vi "ReadBackHNSLogsV2.vi"() -> ()   [LabVIEW 2014]
uses:
  SABL_Source_OLD/HNSCluster.ctl
  SABL_Source_OLD/HNSAI.ctl
  SABL_Source_OLD/HNSWarnings.ctl
  SABL_Source_OLD/HNSMetaCluster.ctl
panel:
  out "appended array":T1[](array[typedef]) {"Overall Status" format="%x"; "PEP Request Word 2" format="%x"; "PEP Request Word 1" format="%x"}
  in  "Array 4":T1[](array[typedef])=array[14302 elements] {"Overall Status" format="%x"; "PEP Request Word 2" format="%x"; "PEP Request Word 1" format="%x"}
  out "Array 3":T2[](array[typedef])
  in  "Array 2":T2[](array[typedef])=array[38192 elements]
  out "Numeric 6":i32
  out "Numeric 5":i32
  out "status 2":bool
  out "Numeric 4":i32
  out "length 2":i32
  in  "HNSLog-2016-02-24-13-03-37.log":T2[](array[typedef])=array[25394 elements]
  out "length":i32
  out "status":bool
  out "Numeric 3":i32
  out "Array":T2[](array[typedef])
  out "transposed array":dbl[][](array[numeric])
  out "Number of Files":i32
  out "All Files in Dir":path[](array[path])
  out "Numeric 2":i32
  out "Numeric":i32
  out "Waveform Graph":dbl[][](graph)
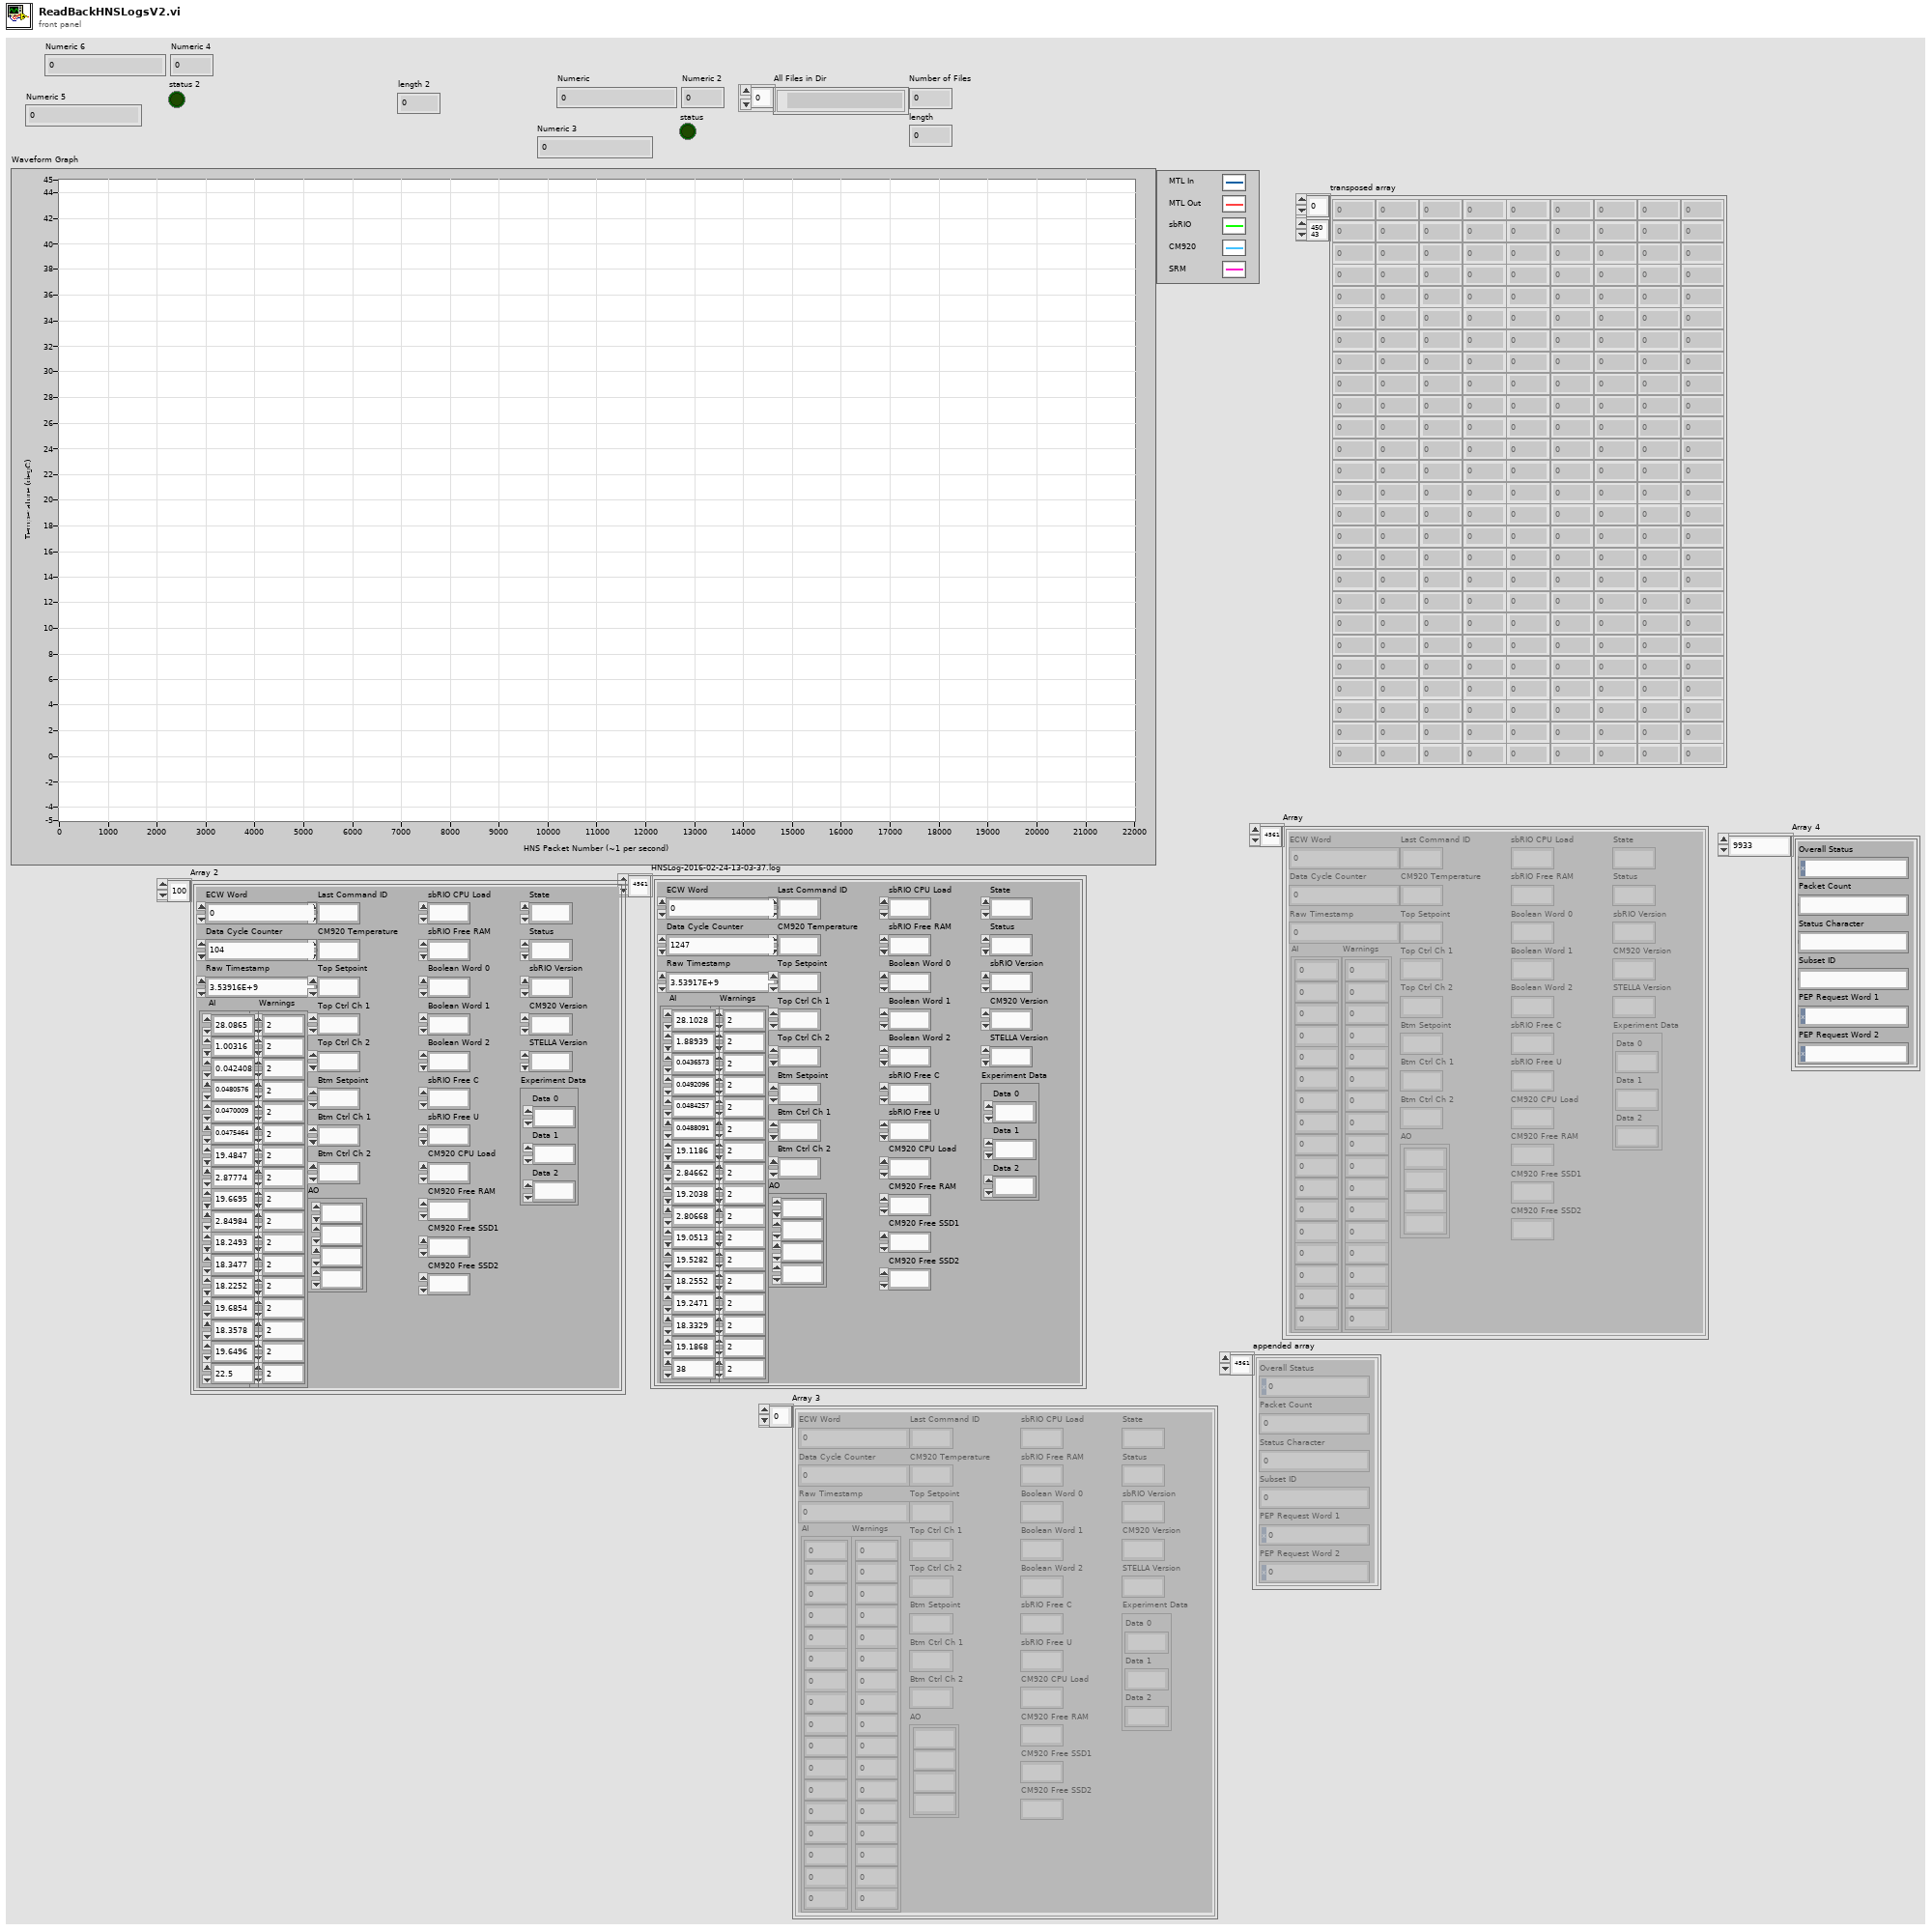
[diagram p1: front panel]
types:
  T1 = typedef "HNSMetaCluster.ctl" = cluster{"Overall Status":u32, "Packet Count":u32, "Status Character":u8, "Subset ID":u16, "PEP Request Word 1":u16, "PEP Request Word 2":u16}
  T2 = typedef "HNSCluster.ctl" = cluster{"ECW Word":u16, "Data Cycle Counter":u16, "Raw Timestamp":dbl, "AI":T3, "Warnings":T4, "Last Command ID":u8, "CM920 Temperature":sgl, "Top Setpoint":sgl, "Top Ctrl Ch 1":i16, "Top Ctrl Ch 2":i16, "Btm Setpoint":sgl, "Btm Ctrl Ch 1":i16, "Btm Ctrl Ch 2":i16, "AO":cluster{sgl, sgl, sgl, sgl}, "sbRIO CPU Load":i16, "sbRIO Free RAM":i16, "Boolean Word 0":i16, "Boolean Word 1":i16, "Boolean Word 2":i16, "sbRIO Free C":i16, "sbRIO Free U":i16, "CM920 CPU Load":i16, "CM920 Free RAM":i16, "CM920 Free SSD1":i16, "CM920 Free SSD2":i16, "State":i16, "Status":i16, "sbRIO Version":sgl, "CM920 Version":sgl, "STELLA Version":sgl, "Experiment Data":cluster{"Data 0":sgl, "Data 1":sgl, "Data 2":sgl}}
  T3 = typedef "HNSAI.ctl" = cluster{"AI0 - Payload Voltage":sgl, "AI1 - Payload Current":sgl, "AI2 - SRM AI1":sgl, "AI3 - SRM AI2":sgl, "AI4 - SRM AI3":sgl, "AI5 - SRM AI4":sgl, "AI6 - Top Back Temp":sgl, "AI7 - Top TEC Current":sgl, "AI8 - Btm Back Temp":sgl, "AI9 - Btm TEC Current":sgl, "AI10 - MTL In Temp":sgl, "AI11 - MTL Out Temp":sgl, "AI12 - Top HX Temp":sgl, "AI13 - Top Front Temp":sgl, "AI14 - Btm HX Temp":sgl, "AI15 - Btm Front Temp":sgl, "AIBT - sbRIO Temp":sgl}
  T4 = typedef "HNSWarnings.ctl" = cluster{"AI0 Warning - Payload Voltage":i8, "AI1 Warning- Payload Current":i8, "AI2 Warning - SRM AI1":i8, "AI3 Warning - SRM AI2":i8, "AI4 Warning - SRM AI3":i8, "AI5 Warning - SRM AI4":i8, "AI6 Warning - Top Back Temp":i8, "AI7 Warning - Top TEC Current":i8, "AI 8 Warning - Btm Back Temp":i8, "AI9 Warning - Btm TEC Current":i8, "AI10 Warning - MTL In Temp":i8, "AI11 Warning - MTL Out Temp":i8, "AI12 Warning - Top HX Temp":i8, "AI13 Warning - Top Front Temp":i8, "AI14 Warning - Btm HX Temp":i8, "AI15 Warning - Btm Front Temp":i8, "AIBT Warning - sbRIO Temp":i8}
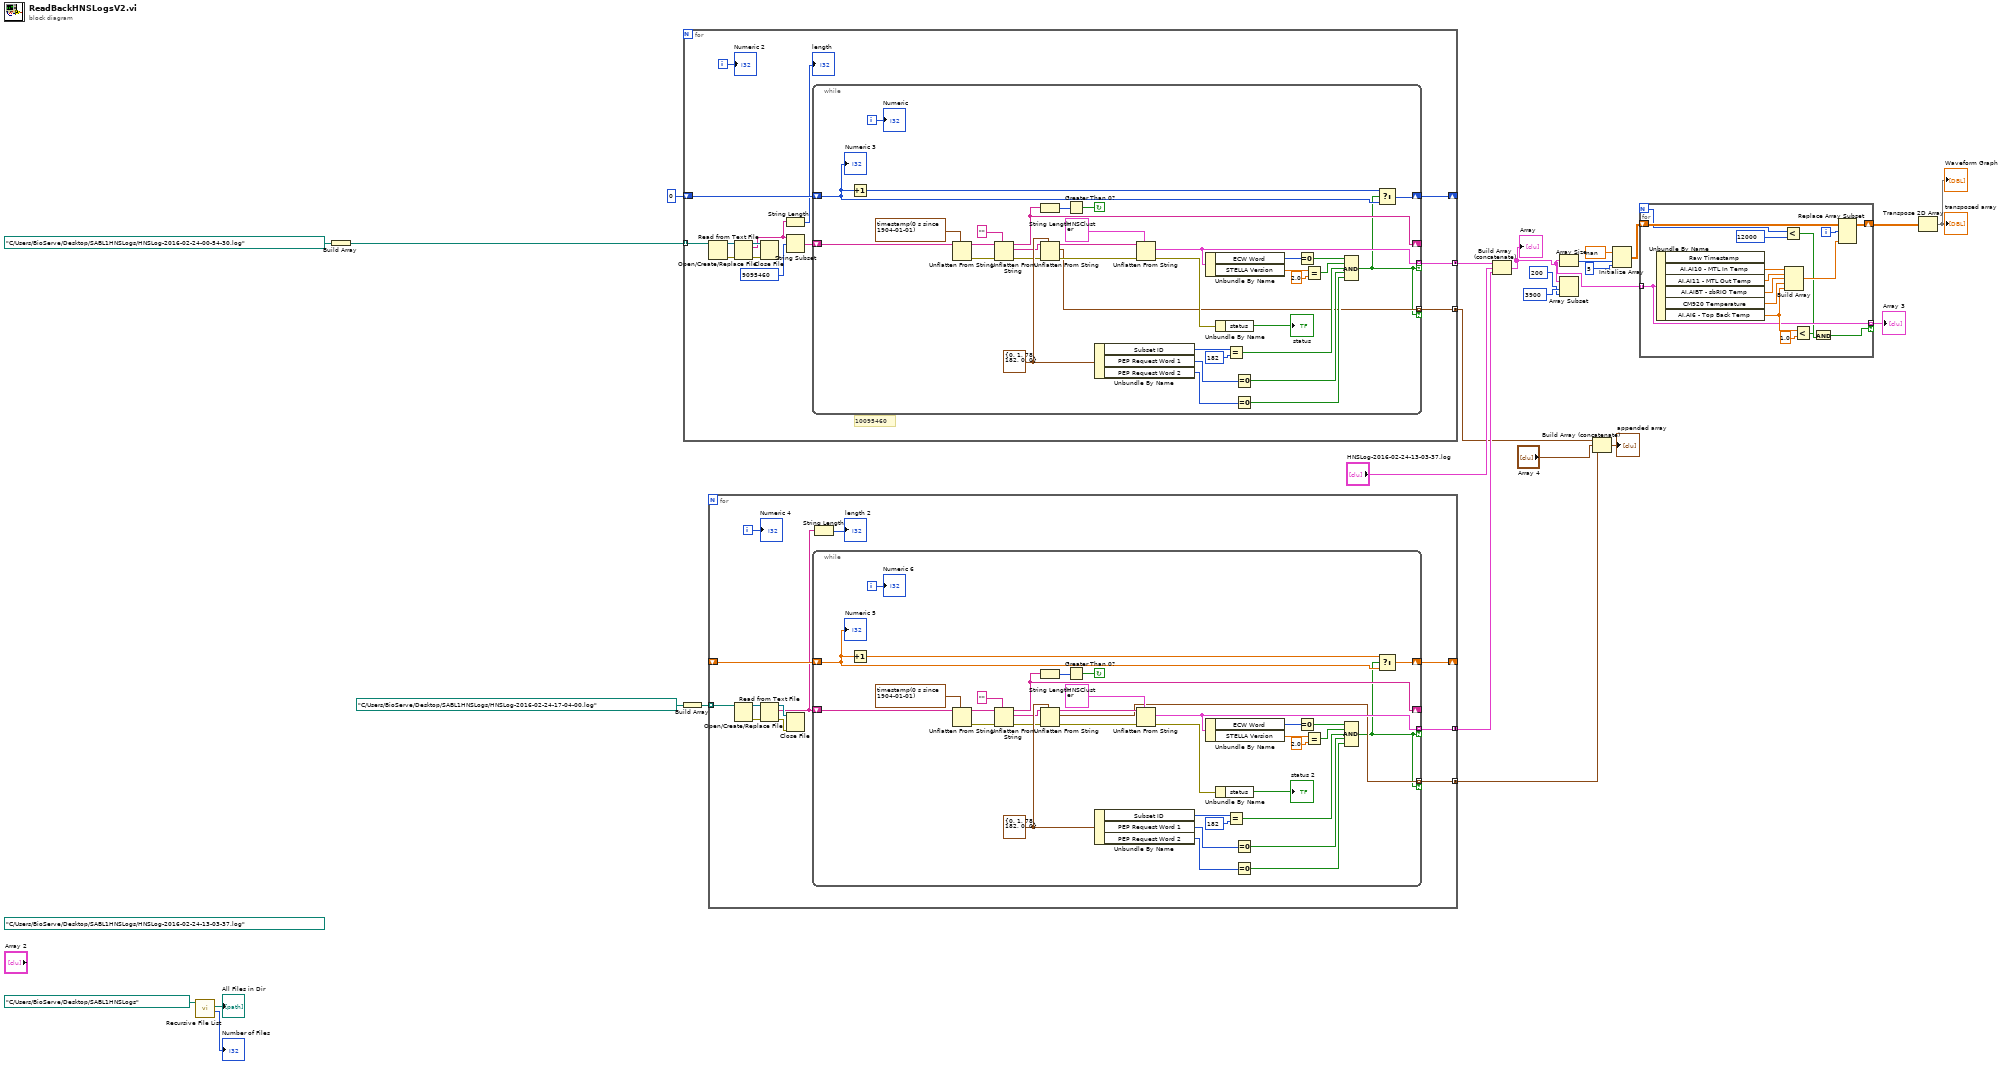
[diagram p0: block diagram]
diagram:
  (unwired) path "C:/Users/BioServe/Desktop/SABL1HNSLogs/HNSLog-2016-02-24-13-03-37.log" ("Folder Path")
  n1 = call <vilib>:"Recursive File List.vi"("Folder Path"=path "C:/Users/BioServe/Desktop/SABL1HNSLogs") -> ("Number of Files"=→"Number of Files":i32, "All Files in Dir"=→"All Files in Dir":path[])  [unwired: 6 in, 3 out]
  n2 = Build Array(path "C:/Users/BioServe/Desktop/SABL1HNSLogs/HNSLog-2016-02-24-00-54-30.log" ("Folder Path")) -> (w15:path[])
  n3 = for {
    tunnel: w15 -> [w31] mode=indexing
    tunnel: [w34] -> w13 mode=concatenating
    shift-right: [w32] -> _
    shift-left: 0 -> [w33]
    tunnel: [w26] -> w5 mode=concatenating
    i -> [w35]
    # "10095460"
    n4 = Open/Create/Replace File(file path (use dialog)=w31) -> (refnum out=w39:refnum<file>, error out=w38:errorcluster)  [unwired: 5 in, 1 out]
    n5 = Read from Text File(file (use dialog)=w39, error in=w38) -> (refnum out=w36:refnum<file>, text=w29:string, error out=w37:errorcluster)  [unwired: 2 in, 1 out]
    n6 = Close File(refnum=w36, error in=w37) -> ()  [unwired: 2 out]
    n7 = String Length(string=w29) -> (length=→"length":i32)
    n8 = String Subset(string=w29, offset (0)=9095460) -> (substring=w28:string)  [unwired: 1 in]
    n9 = while {
      tunnel: [w71] -> w34 mode=indexing if=w40
      shift-right: [w42] -> _
      shift-left: w28 -> [w54]
      shift-right: [w63] -> w32
      shift-left: w33 -> [w64]
      tunnel: [w41] -> w26 mode=indexing if=w40
      i -> [w73]
      stop <- w66 continue-if-true
      w62 = T1 {"Overall Status"=0, "Packet Count"=1, "Status Character"=78, "Subset ID"=182, "PEP Request Word 1"=0, "PEP Request Word 2"=0} ("HNS Meta Cluster")
      n10 = Increment(x=w64) -> (x+1=w65:i32)
      n11 = Unflatten From String(type=timestamp(0 s since 1904-01-01), binary string=w54) -> (rest of the binary string=w47:string, error out=w45:errorcluster)  [unwired: 3 in, 1 out]
      n12 = Unflatten From String(type="", binary string=w47, error in (no error)=w45) -> (rest of the binary string=w42:string, value=w46:string, error out=w44:errorcluster)  [unwired: 2 in]
      n13 = String Length(string=w42) -> (length=w67:i32)
      n14 = Unflatten From String(type=w62, binary string=w46, error in (no error)=w44) -> (rest of the binary string=w72:string, value=w41:T1, error out=w43:errorcluster)  [unwired: 2 in]
      n15 = Greater Than 0?(x=w67) -> (x > 0?=w66:bool)
      n16 = Unbundle By Name(w62) -> ("Subset ID"=w61:u16, "PEP Request Word 1"=w58:u16, "PEP Request Word 2"=w55:u16)
      n17 = Unflatten From String(type=T2 {"ECW Word"=0, "Data Cycle Counter"=0, "Raw Timestamp"=0.0, "AI"={"AI0 - Payload Voltage"=0.0, "AI1 - Payload Current"=0.0, "AI2 - SRM AI1"=0.0, "AI3 - SRM AI2"=0.0, "AI4 - SRM AI3"=0.0, "AI5 - SRM AI4"=0.0, "AI6 - Top Back Temp"=0.0, "AI7 - Top TEC Current"=0.0, "AI8 - Btm Back Temp"=0.0, "AI9 - Btm TEC Current"=0.0, "AI10 - MTL In Temp"=0.0, "AI11 - MTL Out Temp"=0.0, "AI12 - Top HX Temp"=0.0, "AI13 - Top Front Temp"=0.0, "AI14 - Btm HX Temp"=0.0, "AI15 - Btm Front Temp"=0.0, "AIBT - sbRIO Temp"=0.0}, "Warnings"={"AI0 Warning - Payload Voltage"=0, "AI1 Warning- Payload Current"=0, "AI2 Warning - SRM AI1"=0, "AI3 Warning - SRM AI2"=0, "AI4 Warning - SRM AI3"=0, "AI5 Warning - SRM AI4"=0, "AI6 Warning - Top Back Temp"=0, "AI7 Warning - Top TEC Current"=0, "AI 8 Warning - Btm Back Temp"=0, "AI9 Warning - Btm TEC Current"=0, "AI10 Warning - MTL In Temp"=0, "AI11 Warning - MTL Out Temp"=0, "AI12 Warning - Top HX Temp"=0, "AI13 Warning - Top Front Temp"=0, "AI14 Warning - Btm HX Temp"=0, "AI15 Warning - Btm Front Temp"=0, "AIBT Warning - sbRIO Temp"=0}, "Last Command ID"=0, "CM920 Temperature"=0.0, "Top Setpoint"=0.0, "Top Ctrl Ch 1"=0, "Top Ctrl Ch 2"=0, "Btm Setpoint"=0.0, "Btm Ctrl Ch 1"=0, "Btm Ctrl Ch 2"=0, "AO"={0.0, 0.0, 0.0, 0.0}, "sbRIO CPU Load"=0, "sbRIO Free RAM"=0, "Boolean Word 0"=0, "Boolean Word 1"=0, "Boolean Word 2"=0, "sbRIO Free C"=0, "sbRIO Free U"=0, "CM920 CPU Load"=0, "CM920 Free RAM"=0, "CM920 Free SSD1"=0, "CM920 Free SSD2"=0, "State"=0, "Status"=0, "sbRIO Version"=0.0, "CM920 Version"=0.0, "STELLA Version"=0.0, "Experiment Data"={"Data 0"=0.0, "Data 1"=0.0, "Data 2"=0.0}} ("HNS Cluster"), binary string=w72, error in (no error)=w43) -> (value=w71:T2, error out=w53:errorcluster)  [unwired: 2 in, 1 out]
      n18 = Unbundle By Name(w71) -> ("ECW Word"=w51:u16, "STELLA Version"=w70:sgl)
      n19 = Unbundle By Name(w53) -> ("status"=→"status":bool)
      n20 = Equal?(x=w61, y=u16 182) -> (x = y?=w59:bool)
      n21 = Equal To 0?(x=w58) -> (x = 0?=w57:bool)
      n22 = Equal To 0?(x=w55) -> (x = 0?=w56:bool)
      n23 = Equal To 0?(x=w51) -> (x = 0?=w50:bool)
      n24 = Equal?(x=w70, y=sgl 2.0) -> (x = y?=w68:bool)
      n25 = Compound Arithmetic op=AND(w50, w68, w59, w57, w56) -> (w40:bool)
      n26 = Select(t=w65, s=w40, f=w64) -> (s? t:f=w63:i32)
      "Numeric" <- w73
      "Numeric 3" <- w64
    }
    "Numeric 2" <- w35
  }
  n27 = Build Array(path "C:/Users/BioServe/Desktop/SABL1HNSLogs/HNSLog-2016-02-24-17-04-00.log" ("Folder Path")) -> (w10:path[])
  n28 = for {
    tunnel: w10 -> [w78] mode=indexing
    tunnel: [w81] -> w9 mode=concatenating
    shift-right: [w79] -> _
    shift-left: _ -> [w80]
    tunnel: [w75] -> w3 mode=concatenating
    i -> [w82]
    n29 = Open/Create/Replace File(file path (use dialog)=w78) -> (refnum out=w86:refnum<file>, error out=w85:errorcluster)  [unwired: 5 in, 1 out]
    n30 = Read from Text File(file (use dialog)=w86, error in=w85) -> (refnum out=w83:refnum<file>, text=w77:string, error out=w84:errorcluster)  [unwired: 2 in, 1 out]
    n31 = Close File(refnum=w83, error in=w84) -> ()  [unwired: 2 out]
    n32 = while {
      tunnel: [w118] -> w81 mode=indexing if=w87
      shift-right: [w89] -> _
      shift-left: w77 -> [w101]
      shift-right: [w110] -> w79
      shift-left: w80 -> [w111]
      tunnel: [w88] -> w75 mode=indexing if=w87
      i -> [w120]
      stop <- w113 continue-if-true
      w109 = T1 {"Overall Status"=0, "Packet Count"=1, "Status Character"=78, "Subset ID"=182, "PEP Request Word 1"=0, "PEP Request Word 2"=0} ("HNS Meta Cluster")
      n33 = Increment(x=w111) -> (x+1=w112:dbl)
      n34 = Unflatten From String(type=timestamp(0 s since 1904-01-01), binary string=w101) -> (rest of the binary string=w94:string, error out=w92:errorcluster)  [unwired: 3 in, 1 out]
      n35 = Unflatten From String(type="", binary string=w94, error in (no error)=w92) -> (rest of the binary string=w89:string, value=w93:string, error out=w91:errorcluster)  [unwired: 2 in]
      n36 = String Length(string=w89) -> (length=w114:i32)
      n37 = Unflatten From String(type=w109, binary string=w93, error in (no error)=w91) -> (rest of the binary string=w119:string, value=w88:T1, error out=w90:errorcluster)  [unwired: 2 in]
      n38 = Greater Than 0?(x=w114) -> (x > 0?=w113:bool)
      n39 = Unbundle By Name(w109) -> ("Subset ID"=w108:u16, "PEP Request Word 1"=w105:u16, "PEP Request Word 2"=w102:u16)
      n40 = Unflatten From String(type=T2 {"ECW Word"=0, "Data Cycle Counter"=0, "Raw Timestamp"=0.0, "AI"={"AI0 - Payload Voltage"=0.0, "AI1 - Payload Current"=0.0, "AI2 - SRM AI1"=0.0, "AI3 - SRM AI2"=0.0, "AI4 - SRM AI3"=0.0, "AI5 - SRM AI4"=0.0, "AI6 - Top Back Temp"=0.0, "AI7 - Top TEC Current"=0.0, "AI8 - Btm Back Temp"=0.0, "AI9 - Btm TEC Current"=0.0, "AI10 - MTL In Temp"=0.0, "AI11 - MTL Out Temp"=0.0, "AI12 - Top HX Temp"=0.0, "AI13 - Top Front Temp"=0.0, "AI14 - Btm HX Temp"=0.0, "AI15 - Btm Front Temp"=0.0, "AIBT - sbRIO Temp"=0.0}, "Warnings"={"AI0 Warning - Payload Voltage"=0, "AI1 Warning- Payload Current"=0, "AI2 Warning - SRM AI1"=0, "AI3 Warning - SRM AI2"=0, "AI4 Warning - SRM AI3"=0, "AI5 Warning - SRM AI4"=0, "AI6 Warning - Top Back Temp"=0, "AI7 Warning - Top TEC Current"=0, "AI 8 Warning - Btm Back Temp"=0, "AI9 Warning - Btm TEC Current"=0, "AI10 Warning - MTL In Temp"=0, "AI11 Warning - MTL Out Temp"=0, "AI12 Warning - Top HX Temp"=0, "AI13 Warning - Top Front Temp"=0, "AI14 Warning - Btm HX Temp"=0, "AI15 Warning - Btm Front Temp"=0, "AIBT Warning - sbRIO Temp"=0}, "Last Command ID"=0, "CM920 Temperature"=0.0, "Top Setpoint"=0.0, "Top Ctrl Ch 1"=0, "Top Ctrl Ch 2"=0, "Btm Setpoint"=0.0, "Btm Ctrl Ch 1"=0, "Btm Ctrl Ch 2"=0, "AO"={0.0, 0.0, 0.0, 0.0}, "sbRIO CPU Load"=0, "sbRIO Free RAM"=0, "Boolean Word 0"=0, "Boolean Word 1"=0, "Boolean Word 2"=0, "sbRIO Free C"=0, "sbRIO Free U"=0, "CM920 CPU Load"=0, "CM920 Free RAM"=0, "CM920 Free SSD1"=0, "CM920 Free SSD2"=0, "State"=0, "Status"=0, "sbRIO Version"=0.0, "CM920 Version"=0.0, "STELLA Version"=0.0, "Experiment Data"={"Data 0"=0.0, "Data 1"=0.0, "Data 2"=0.0}} ("HNS Cluster"), binary string=w119, error in (no error)=w90) -> (value=w118:T2, error out=w100:errorcluster)  [unwired: 2 in, 1 out]
      n41 = Unbundle By Name(w118) -> ("ECW Word"=w98:u16, "STELLA Version"=w117:sgl)
      n42 = Unbundle By Name(w100) -> ("status"=→"status 2":bool)
      n43 = Equal?(x=w108, y=u16 182) -> (x = y?=w106:bool)
      n44 = Equal To 0?(x=w105) -> (x = 0?=w104:bool)
      n45 = Equal To 0?(x=w102) -> (x = 0?=w103:bool)
      n46 = Equal To 0?(x=w98) -> (x = 0?=w97:bool)
      n47 = Equal?(x=w117, y=sgl 2.0) -> (x = y?=w115:bool)
      n48 = Compound Arithmetic op=AND(w97, w115, w106, w104, w103) -> (w87:bool)
      n49 = Select(t=w112, s=w87, f=w111) -> (s? t:f=w110:dbl)
      "Numeric 6" <- w120
      "Numeric 5" <- w111
    }
    n50 = String Length(string=w77) -> (length=→"length 2":i32)
    "Numeric 4" <- w82
  }
  n51 = Build Array (concatenate)(w13, "HNSLog-2016-02-24-13-03-37.log", w9) -> (w1:T2[])
  "Array" <- w1
  n52 = Array Size(array=w1) -> (size(s)=w21:i32)
  n53 = Array Subset(array=w1, index=3900 ("length"), length=200 ("index")) -> ()  [unwired: 1 out]
  n54 = Build Array (concatenate)(w5, "Array 4", w3) -> (→"appended array":T1[])
  n55 = Initialize Array(nan, w21, 5 ("dimension size")) -> (w19:dbl[][])
  n56 = for {
    N -> [w126]
    tunnel: w1 -> [w127] mode=indexing
    shift-right: [w130] -> w18
    shift-left: w19 -> [w133]
    tunnel: [w127] -> w8 mode=indexing if=w122
    i -> [w132]
    n57 = Unbundle By Name(w127) -> ("AI.AI10 - MTL In Temp"=w137:sgl, "AI.AI11 - MTL Out Temp"=w136:sgl, "AI.AIBT - sbRIO Temp"=w135:sgl, "CM920 Temperature"=w134:sgl, "AI.AI6 - Top Back Temp"=w129:sgl)  [unwired: 1 out]
    n58 = Less?(x=w126, y=12000) -> (x < y?=w124:bool)
    n59 = Build Array(w137, w136, w135, w134, w129) -> (w131:sgl[])
    n60 = Less?(x=w129, y=sgl 1.0) -> (x < y?=w123:bool)
    n61 = And(x=w123, y=w124) -> (x .and. y?=w122:bool)
    n62 = Replace Array Subset(array=w133, new element=w131, index (row)=w132) -> (w130:dbl[][])  [unwired: 1 in]
  }
  "Array 3" <- w8
  n63 = Transpose 2D Array(2D array=w18) -> (transposed array=→"Waveform Graph" →"transposed array":dbl[][])
